vi "kim - read m file.vi"(0 "file path":path=path "\\\\rus-one\\newdata/data/Ultrasound/Experiment/ProbeTest/Probe10/Hg1201-6-C185-550Cair-3c-83K/sweep3/9w/3366_a.dat") -> (4 "Temperature (K) Array":dbl[](array[numeric]), 6 "Frequency (kHz) Array":dbl[](array[numeric]), 8 "OK?":bool, 10 "Gamma (kHz) Array":dbl[](array[numeric]), 14 "time (min)":dbl[](array[numeric]), 15 "Field (T) Array":dbl[](array[numeric]))   [LabVIEW 2015]
uses:
  <vilib>/Utility/file.llb/Read From Spreadsheet File (string).vi
  <vilib>/regexp/Match Regular Expression.xnode
panel:
  in  "error IO":errorcluster
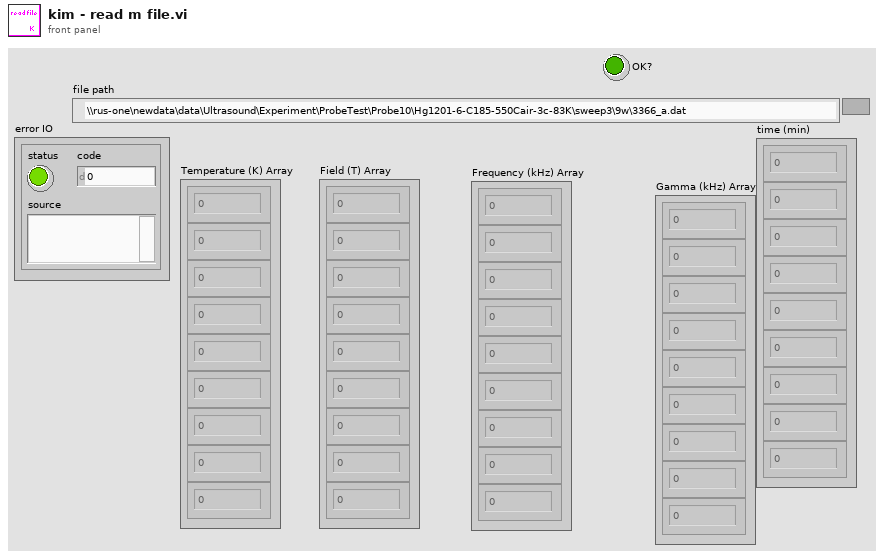
[diagram p1: front panel]
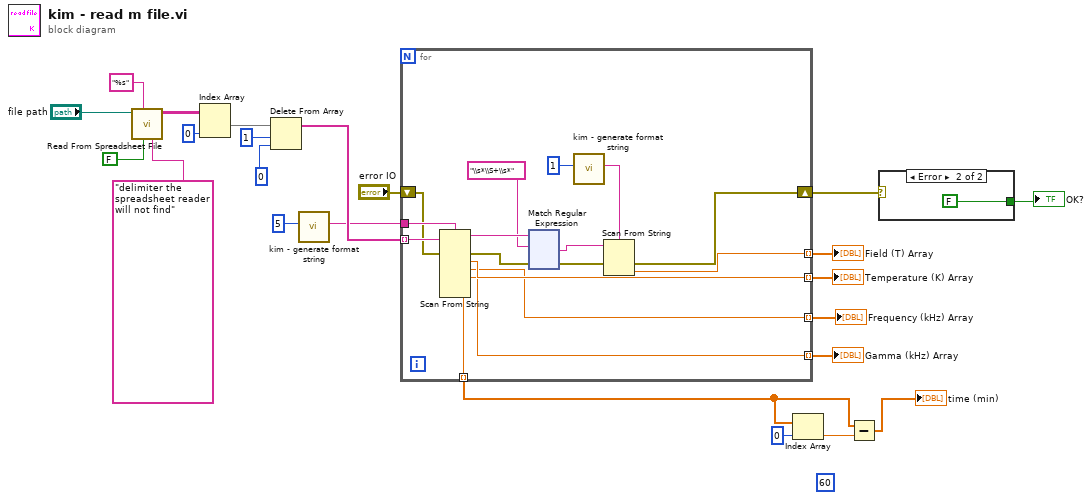
[diagram p0: block diagram]
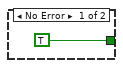
[diagram p2: hidden frame]
diagram:
  (unwired) 60 ("index")
  n1 = call-poly <vilib>:"Read From Spreadsheet File.vi"("delimiter (\\t)"="delimiter the spreadsheet reader will not find" ("delimiter (\\t)"), "transpose (no:F)"=FALSE ("append to file? (new file:F)"), "format (%s)"="%s", "file path (dialog if empty)"="file path") -> ("all rows"=w21:string[][])  [unwired: 3 in, 4 out]
  n2 = Index Array(array=w21, index (col)=0 ("disabled index (col)")) -> (element=w19:string[])  [unwired: 1 in]
  n3 = Delete From Array(array=w19, length=1, index=0) -> (array with subset deleted=w14:string[])  [unwired: 1 out]
  n4 = call "kim - generate format string.vi"("number"=5) -> ("format"=w12:string)  [unwired: 10 in]
  n5 = for {
    tunnel: w14 -> [w29] mode=indexing
    tunnel: w12 -> [w38]
    tunnel: [w33] -> w11 mode=indexing
    tunnel: [w32] -> w10 mode=indexing
    tunnel: [w31] -> w9 mode=indexing
    tunnel: [w30] -> w8 mode=indexing
    shift-right: [w26] -> w6
    shift-left: "error IO" -> [w25]
    tunnel: [w24] -> w3 mode=indexing
    n6 = Scan From String(format string=w38, input string=w29, error in=w25) -> (remaining string=w39:string, error out=w28:errorcluster, output 1=w33:dbl, output 2=w31:dbl, output 3=w30:dbl, output 5=w24:dbl)  [unwired: 7 in, 1 out]
    n7 = xnode "Match Regular Expression"("input string"=w39, "regular expression"="\\s*\\S+\\s*", "error in"=w28) -> ("after match"=w36:string, "error out"=w27:errorcluster)  [unwired: 3 in, 3 out]
    n8 = call "kim - generate format string.vi"("number"=1) -> ("format"=w34:string)  [unwired: 10 in]
    n9 = Scan From String(format string=w34, input string=w36, error in=w27) -> (error out=w26:errorcluster, output 1=w32:dbl)  [unwired: 2 in, 2 out]
  }
  "Temperature (K) Array" <- w11
  "Field (T) Array" <- w10
  "Frequency (kHz) Array" <- w9
  "Gamma (kHz) Array" <- w8
  n10 = Index Array(array=w3, index=0) -> (element=w2:dbl)
  n11 = Subtract(x=w3, y=w2) -> (x-y=→"time (min)":dbl[])
  n12 = case shown="Error" w6 {
    tunnel: [TRUE FALSE] -> w5
    frame No Error {
    }
    frame Error {
    }
  }
  "OK?" <- w5
